vi "SiosIfmSensorProperty.vi"(0 "Device Number":i32, 1 "Sensor":i32(knob) scale=1.0..24.0) -> (2 "Output Value":u32, 3 "Channel":u32 format="%b", 4 "Type":u32, 5 "corr on/off":u32)   [LabVIEW 2009]
uses:
  siosifm.dll
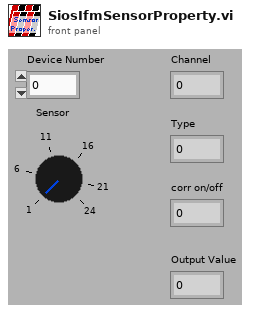
[diagram p1: front panel]
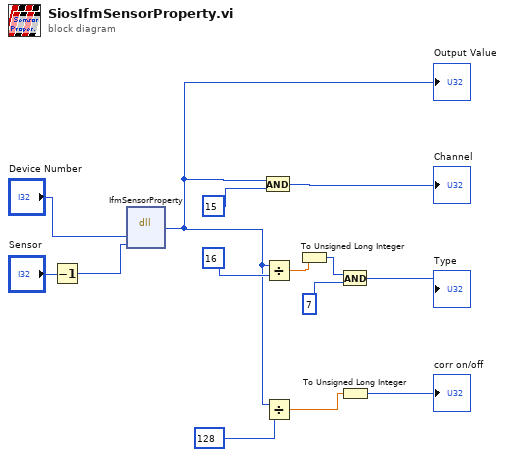
[diagram p0: block diagram]
diagram:
  n1 = Decrement(x="Sensor") -> (x-1=w13:i32)
  n2 = dll-call lib="C:/WORK/Artem/RE-10/SIOS_IfmDLL/siosifm.dll" fn="IfmSensorProperty"("devNumber"="Device Number", "Sensor"=w13) -> ("value"=w5:u32)  [unwired: 5 in, 2 out]
  "Output Value" <- w5
  n3 = And(x=w5, y=u32 15) -> (x .and. y?=→"Channel":u32)
  n4 = Divide(x=w5, y=u32 16) -> (x/y=w1:dbl)
  n5 = Divide(x=w5, y=u32 128) -> (x/y=w8:dbl)
  n6 = To Unsigned Long Integer(number=w1) -> (unsigned 32bit integer=w2:u32)
  n7 = And(x=w2, y=u32 7) -> (x .and. y?=→"Type":u32)
  n8 = To Unsigned Long Integer(number=w8) -> (unsigned 32bit integer=→"corr on/off":u32)
